vi "Unsupported Type.vi"() -> ()   [LabVIEW 2017, in "Assertions.Tests.lvlib" / "Assert Count.lvlib"]
uses:
  Assert Count.lvlib
  src/Transparent Assertions/Assertions/Assertions.lvlib
panel:
  out "error out":errorcluster
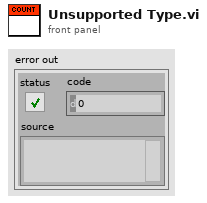
[diagram p1: front panel]
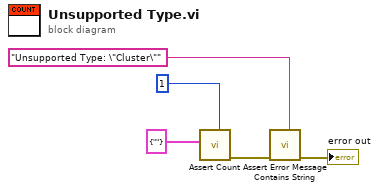
[diagram p0: block diagram]
diagram:
  n1 = call "Assert Count.vi"("Expected"=1, "Haystack"=cluster{string} {""}) -> ("error out"=w3:errorcluster)  [unwired: 9 in]
  n2 = call "Assert Error Message Contains String.vi"("Expected"="Unsupported Type: \"Cluster\"", "error in (no error)"=w3) -> ("error out"=→"error out":errorcluster)  [unwired: 9 in]
